vi "Read ADC.vi"(8 "error in (no error)":errorcluster, 10 "canal":dbl, 11 "NXP in":refnum<class "NXP.lvclass">) -> (0 "error out":errorcluster, 3 "NXP out":refnum<class "NXP.lvclass">)   [LabVIEW 2019, in "NXP.lvclass"]
uses:
  NXP.lvclass
  NXP.lvclass/NXP.ctl
  d6bdf711-9eee-4e02-ab25-74ba970acb71.vi
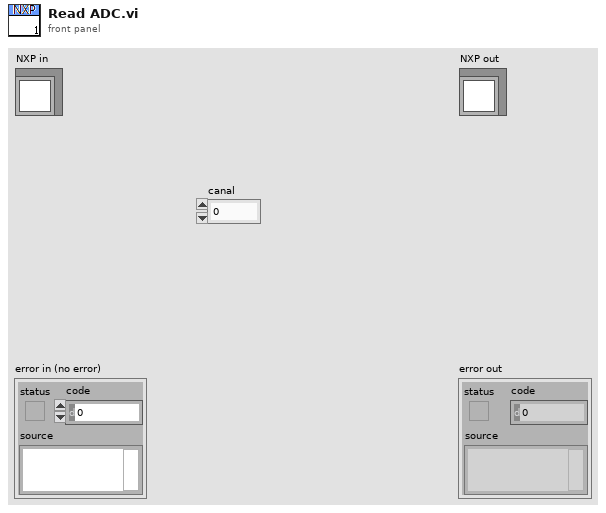
[diagram p1: front panel]
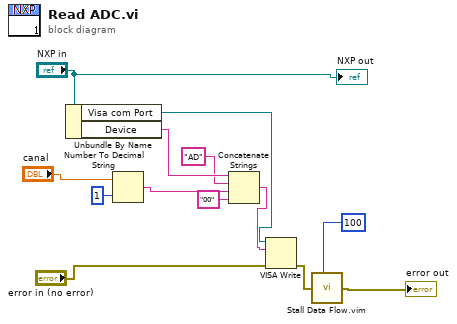
[diagram p0: block diagram]
diagram:
  n1 = Unbundle By Name("NXP in") -> ("Visa com Port"=w5:refnum<visa-resource-name>, "Device"=w10:string)
  n2 = Number To Decimal String(number="canal", width (-)=i16 1) -> (decimal integer string=w8:string)
  n3 = Concatenate Strings(w10, "AD" ("string"), w8, "00" ("string")) -> (w6:string)
  n4 = VISA Write(VISA resource name=w5, write buffer=w6, error in (no error)="error in (no error)") -> (error out=w4:errorcluster)  [unwired: 2 out]
  n5 = call "Stall Data Flow.vim"("value in"=w4, "milliseconds to wait"=u32 100) -> ("value out"=→"error out":errorcluster)  [unwired: 1 out]
  "NXP out" <- "NXP in"
